vi "Object Tester.vi"() -> ()   [LabVIEW 2025, in "Power Supply.lvlib" / "generic-power-supply.lvclass"]
uses:
  generic-power-supply/generic-power-supply.lvclass
  hardware-selection.ctl
  <vilib>/Handler Framework/CmdQueue/Enqueue Single.vi
  PSP-603/PSP-603.lvclass
  generic-power-supply/generic-power-supply.lvclass/generic-power-supply.ctl
  <vilib>/Handler Framework/Handler Framework.lvlib
  C:/Users/grove/Desktop/LabVIEW/Git/dqmh-lvoop-template/Libraries/Power Supply/Classes/generic-power-supply/generic-power-supply.lvclass
  C:/Users/grove/Desktop/LabVIEW/Git/dqmh-lvoop-template/Libraries/Power Supply/Classes/PSP-603/PSP-603.lvclass
panel:
  out "error out":errorcluster
  in  "Tab Control":enum32{"Set Output"}(tab)
  in  "Current":dbl=0.05
  in  "Set Voltage":bool
  in  "Voltage":dbl=10.0
  in  "Set Current":bool
  in  "Output":bool
  out "Voltage [V]":dbl format="%_4g"
  in  "Read Voltage":bool
  in  "Read Current":bool
  out "Current [A]":dbl format="%_4g"
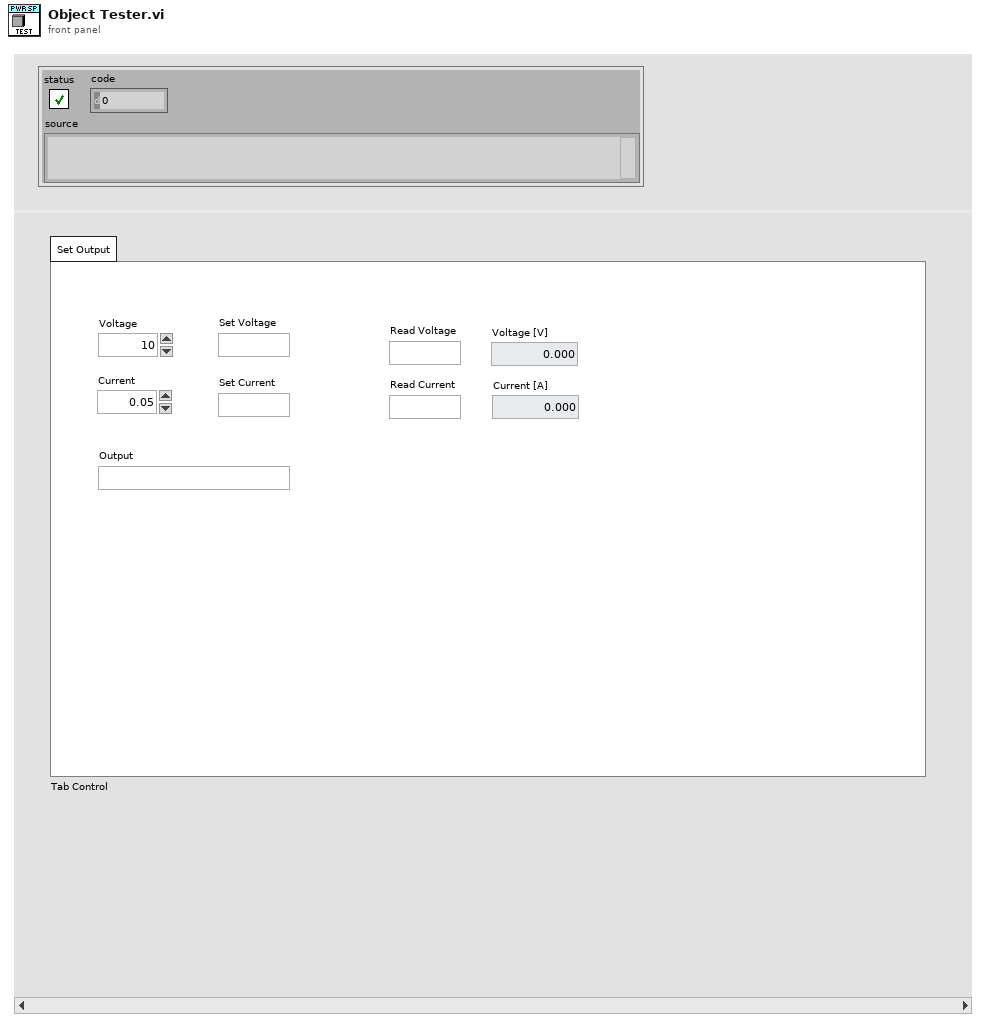
[diagram p1: front panel]
types:
  T1 = typedef "hardware-selection.ctl" = enum16{"Parent", "Simulation", "PSP-603"}
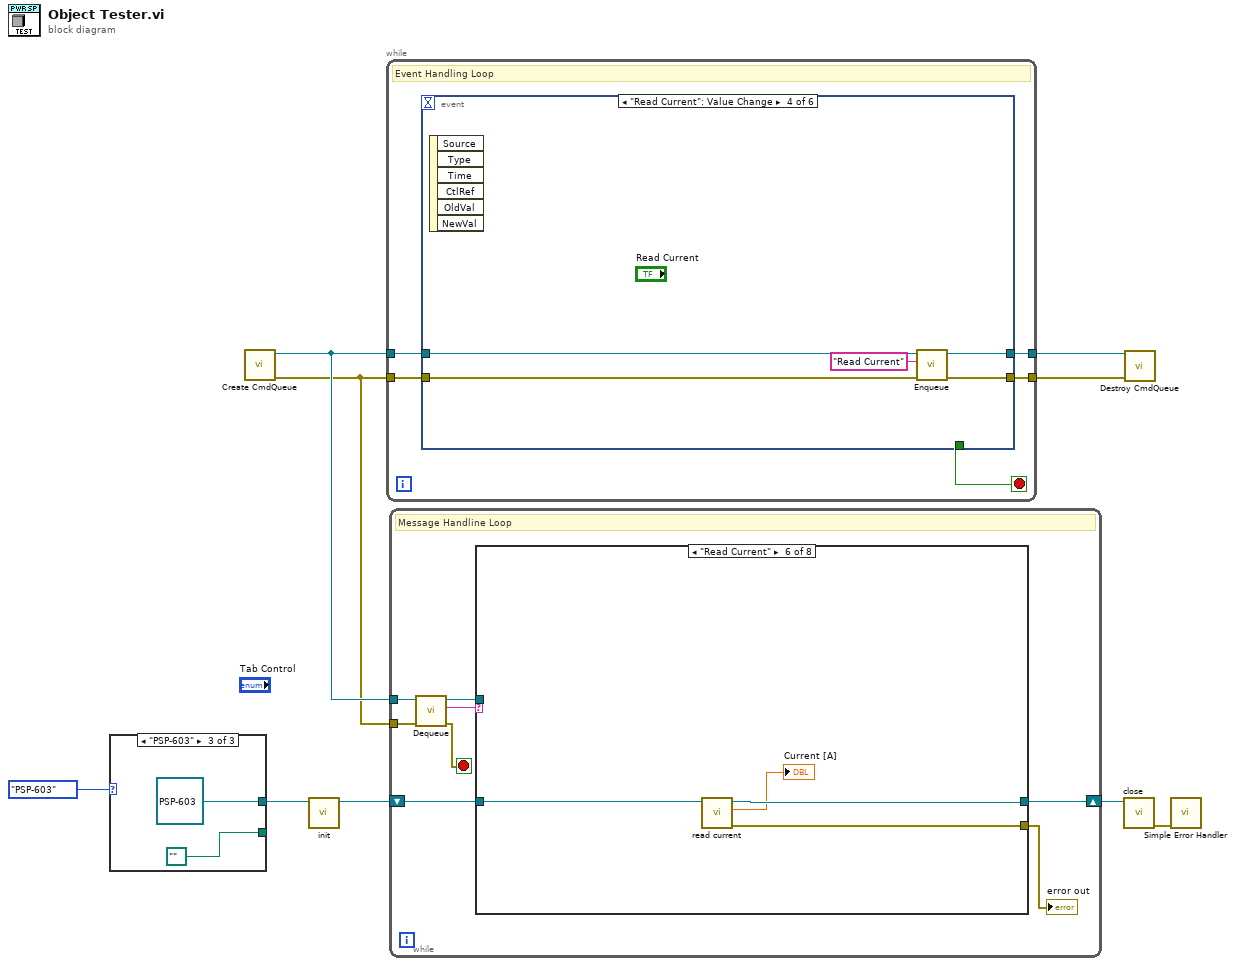
[diagram p0: block diagram]
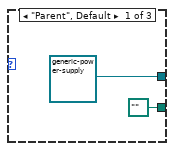
[diagram p2: hidden frame]
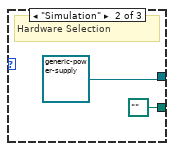
[diagram p3: hidden frame]
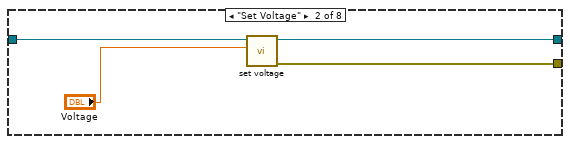
[diagram p5: hidden frame]
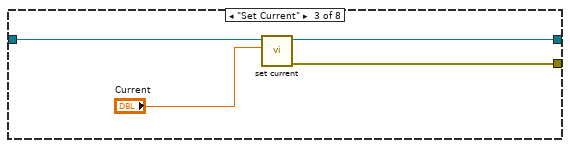
[diagram p6: hidden frame]
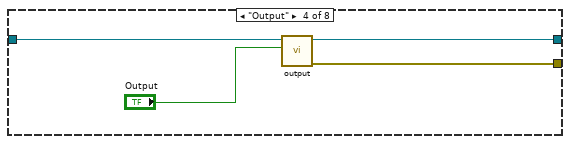
[diagram p7: hidden frame]
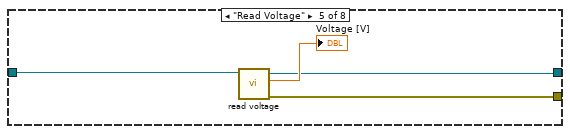
[diagram p8: hidden frame]
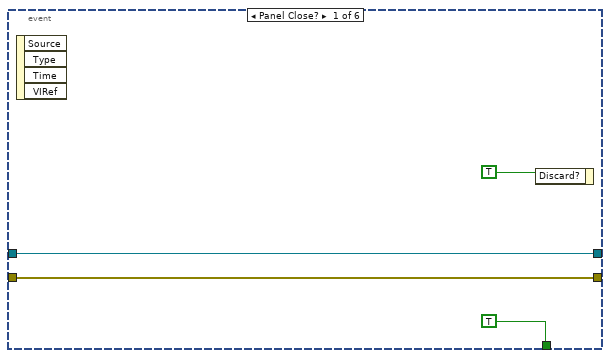
[diagram p11: hidden frame]
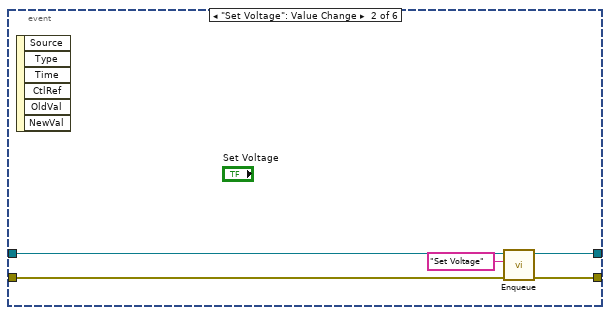
[diagram p12: hidden frame]
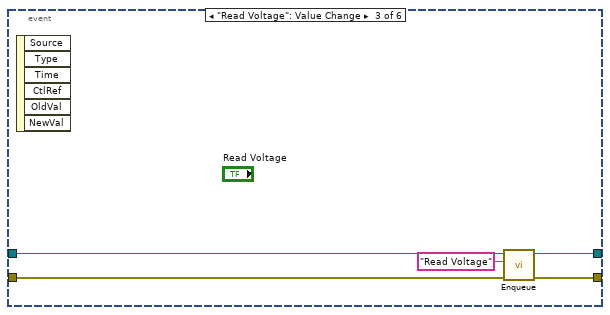
[diagram p13: hidden frame]
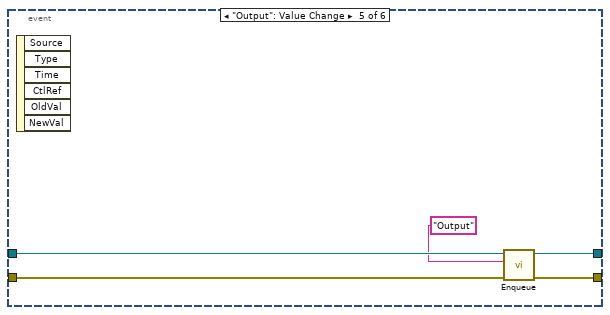
[diagram p14: hidden frame]
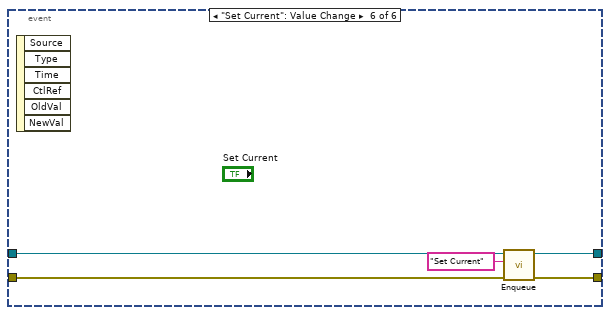
[diagram p15: hidden frame]
diagram:
  n1 = case shown="\"PSP-603\"" hardware-selection."PSP-603" {
    tunnel: [path "" ("Path") path "" ("Path") path "" ("Path")] -> _
    tunnel: [refnum<class "generic-power-supply.lvclass"> refnum ("Power Supply.lvlib:generic-power-supply.lvclass") refnum<class "generic-power-supply.lvclass"> refnum ("Power Supply.lvlib:generic-power-supply.lvclass") refnum<class "PSP-603.lvclass"> refnum ("Power Supply.lvlib:PSP-603.lvclass")] -> w4
    frame "Parent", Default {
    }
    frame "Simulation" {
      # "Hardware Selection"
    }
    frame "PSP-603" {
    }
  }
  n2 = call <vilib>:"Create CmdQueue.vi"() -> ("error out"=w8:errorcluster, "CmdQueue out"=w9:refnum<queue>)  [unwired: 10 in]
  n3 = call-dynamic "init.vi"("generic-power-supply in"=w4) -> ("generic-power-supply out"=w3:refnum<class "generic-power-supply.lvclass">)  [unwired: 9 in, 1 out]
  n4 = while {
    tunnel: w9 -> [w19]
    tunnel: w8 -> [w18]
    tunnel: [w17] -> w7
    tunnel: [w16] -> w6
    stop <- w20 stop-if-true
    # "Event Handling Loop"
    n5 = event shown="[3] \"Read Current\": Value Change" {
      selector: _ -> [_ _ _ _ _ _]
      dyn-events: _ -> [_ _ _ _ _ _]
      timeout: _ -> [_ _ _ _ _ _]
      tunnel: [TRUE _ _ _ _ _] -> w20
      tunnel: w19 -> [w22 w27 w32 w37 w42 w47]
      tunnel: w18 -> [w21 w26 w31 w36 w41 w46]
      tunnel: [w22 w29 w34 w39 w44 w49] -> w17
      tunnel: [w21 w28 w33 w38 w43 w48] -> w16
      event Panel Close? {
        n6 = event-data() -> ()  [unwired: 1 in, 4 out]
        n7 = event-data("Discard?"=TRUE) -> ()  [unwired: 1 in, 1 out]
      }
      event "Set Voltage": Value Change {
        n8 = event-data() -> ()  [unwired: 1 in, 6 out]
        n9 = call-poly <vilib>:"Enqueue.vi"("error in (no error)"=w26, "Command"="Set Voltage", "CmdQueue in"=w27) -> ("error out"=w28:errorcluster, "CmdQueue out"=w29:refnum<queue>)  [unwired: 7 in]
      }
      event "Read Voltage": Value Change {
        n10 = event-data() -> ()  [unwired: 1 in, 6 out]
        n11 = call-poly <vilib>:"Enqueue.vi"("error in (no error)"=w31, "Command"="Read Voltage", "CmdQueue in"=w32) -> ("error out"=w33:errorcluster, "CmdQueue out"=w34:refnum<queue>)  [unwired: 7 in]
      }
      event "Read Current": Value Change {
        n12 = event-data() -> ()  [unwired: 1 in, 6 out]
        n13 = call-poly <vilib>:"Enqueue.vi"("error in (no error)"=w36, "Command"="Read Current", "CmdQueue in"=w37) -> ("error out"=w38:errorcluster, "CmdQueue out"=w39:refnum<queue>)  [unwired: 7 in]
      }
      event "Output": Value Change {
        n14 = event-data() -> ()  [unwired: 1 in, 6 out]
        n15 = call-poly <vilib>:"Enqueue.vi"("error in (no error)"=w41, "Command"="Output", "CmdQueue in"=w42) -> ("error out"=w43:errorcluster, "CmdQueue out"=w44:refnum<queue>)  [unwired: 7 in]
      }
      event "Set Current": Value Change {
        n16 = event-data() -> ()  [unwired: 1 in, 6 out]
        n17 = call-poly <vilib>:"Enqueue.vi"("error in (no error)"=w46, "Command"="Set Current", "CmdQueue in"=w47) -> ("error out"=w48:errorcluster, "CmdQueue out"=w49:refnum<queue>)  [unwired: 7 in]
      }
    }
  }
  n18 = while {
    tunnel: w9 -> [w57]
    tunnel: w8 -> [w56]
    shift-right: [w51] -> w2
    shift-left: w3 -> [w52]
    stop <- w55 stop-if-true
    # "Message Handline Loop"
    n19 = call <vilib>:"Dequeue.vi"("error in (no error)"=w56, "CmdQueue in"=w57) -> ("error out"=w55:errorcluster, "cmd"=w54:string, "CmdQueue out"=w53:refnum<queue>)  [unwired: 5 in, 2 out]
    n20 = case shown="\"Read Current\"" w54 {
      tunnel: w53 -> [_ _ _ _ _ _ _ _]
      tunnel: w52 -> [w58 w62 w66 w70 w74 w78 w79 w80]
      tunnel: [w58 w61 w65 w68 w72 w77 w79 w80] -> w51
      tunnel: [_ w59 w64 w67 w71 w76 _ _] -> w50
      frame Default {
      }
      frame "Set Voltage" {
        n21 = call-dynamic "set voltage.vi"("Voltage"="Voltage", "generic-power-supply in"=w62) -> ("error out"=w59:errorcluster, "generic-power-supply out"=w61:refnum<class "generic-power-supply.lvclass">)  [unwired: 8 in]
      }
      frame "Set Current" {
        n22 = call-dynamic "set current.vi"("Current [A]"="Current", "generic-power-supply in"=w66) -> ("error out"=w64:errorcluster, "generic-power-supply out"=w65:refnum<class "generic-power-supply.lvclass">)  [unwired: 8 in]
      }
      frame "Output" {
        n23 = call-dynamic "output.vi"("Output [on/off]"="Output", "generic-power-supply in"=w70) -> ("error out"=w67:errorcluster, "generic-power-supply out"=w68:refnum<class "generic-power-supply.lvclass">)  [unwired: 8 in]
      }
      frame "Read Voltage" {
        n24 = call-dynamic "read voltage.vi"("generic-power-supply in"=w74) -> ("error out"=w71:errorcluster, "Voltage [V]"=→"Voltage [V]":dbl, "generic-power-supply out"=w72:refnum<class "generic-power-supply.lvclass">)  [unwired: 8 in]
      }
      frame "Read Current" {
        n25 = call-dynamic "read current.vi"("generic-power-supply in"=w78) -> ("error out"=w76:errorcluster, "Current [A]"=→"Current [A]":dbl, "generic-power-supply out"=w77:refnum<class "generic-power-supply.lvclass">)  [unwired: 8 in]
      }
      frame "init" {
      }
      frame "shutdown" {
      }
    }
    "error out" <- w50
  }
  n26 = call-dynamic "close.vi"("generic-power-supply in"=w2) -> ("error out"=w1:errorcluster)  [unwired: 9 in, 1 out]
  n27 = call <vilib>:"Destroy CmdQueue.vi"("error in (no error)"=w6, "CmdQueue in"=w7) -> ()  [unwired: 9 in, 1 out]
  n28 = call <vilib>:"Simple Error Handler.vi"("error in (no error)"=w1) -> ()  [unwired: 4 in, 5 out]
